vi "_Calculate cps All.vi"(1 "Raw Counts":i32[](array[numeric])) -> (0 "Data in cps":dbl[](array[numeric]))   [LabVIEW 2012]
uses:
  _Global Configuration.vi
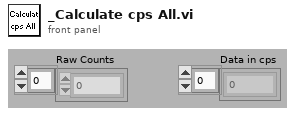
[diagram p1: front panel]
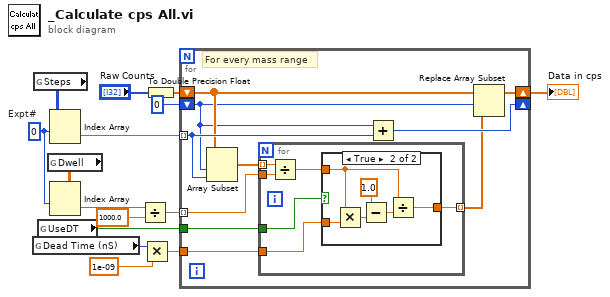
[diagram p0: block diagram]
diagram:
  w11 = 0  # Expt#
  n1 = global read "_Global Configuration.vi" "Dead Time (nS)"() -> (w6:i32)
  n2 = global read "_Global Configuration.vi" "Steps"() -> (w15:i32[][])
  n3 = global read "_Global Configuration.vi" "UseDT"() -> (w1:bool)
  n4 = global read "_Global Configuration.vi" "Dwell"() -> (w12:dbl[][])
  n5 = Index Array(array=w15, index (row)=w11) -> (element=w14:i32[])  [unwired: 1 in]
  n6 = Index Array(array=w12, index (row)=w11) -> (element=w9:dbl[])  [unwired: 1 in]
  n7 = Divide(x=w9, y=1000.0) -> (x/y=w8:dbl[])
  n8 = Multiply(x=w6, y=1e-09) -> (x*y=w5:dbl)
  n9 = To Double Precision Float(number="Raw Counts") -> (double precision float=w4:dbl[])
  n10 = for {
    tunnel: w14 -> [w22] mode=indexing
    shift-right: [w17] -> w2
    shift-left: w4 -> [w20]
    tunnel: w8 -> [w24] mode=indexing
    tunnel: w5 -> [w23]
    shift-right: [w21] -> _
    shift-left: 0 -> [w19]
    tunnel: w1 -> [w16]
    # "For every mass range"
    n11 = Array Subset(array=w20, index=w19, length=w22) -> (w25:dbl[])
    n12 = for {
      tunnel: w24 -> [w31]
      tunnel: w25 -> [w30] mode=indexing
      tunnel: w23 -> [w29]
      tunnel: [w27] -> w18 mode=indexing
      tunnel: w16 -> [w26]
      n13 = Divide(x=w30, y=w31) -> (x/y=w28:dbl)
      n14 = case shown="True" w26 {
        tunnel: w29 -> [_ w38]
        tunnel: w28 -> [w32 w34]
        tunnel: [w32 w33] -> w27
        frame False {
        }
        frame True {
          n15 = Multiply(x=w34, y=w38) -> (x*y=w37:dbl)
          n16 = Subtract(x=1.0 ("y"), y=w37) -> (x-y=w35:dbl)
          n17 = Divide(x=w34, y=w35) -> (x/y=w33:dbl)
        }
      }
    }
    n18 = Add(x=w19, y=w22) -> (x+y=w21:i32)
    n19 = Replace Array Subset(array=w20, new element=w18, index=w19) -> (w17:dbl[])
  }
  "Data in cps" <- w2
